vi "Joystick and Camera SHIH V3.2 - external Connection.vi"(7 "Measurement Point":string, 8 "times per measurement":i32, 9 "Motion in":refnum<class "Motion.lvclass">) -> (0 "error out 2":errorcluster, 2 "final out":dbl[](array[numeric]), 3 "Motion out 2":refnum<class "Motion.lvclass">, 4 "GANTRY position":dbl[](array[numeric]), 5 "radius/stddev":dbl[](array[numeric]))   [LabVIEW 2016]
uses:
  Classes/Controllers/Motion/Copy of Motion Folder/Motion.lvclass
  Classes/Controllers/Camera/Copy of Camera Folder/Machine Vision.ctl
  Classes/Controllers/Camera/Copy of Camera Folder/Camera.lvclass
  Classes/Controllers/Camera/Copy of Controller Folder/Controller.lvclass
panel:
  out "loop index":i32
  out "Radius Standard Dev":dbl
  out "Radius  Mean":dbl
  out "Y Standard Dev":dbl
  out "Y Arithmetic Mean":dbl
  out "X Standard Dev":dbl
  out "X Arithmetic Mean":dbl
  out "camera R":dbl
  out "Image 2":T1(plugin-control)
  out "Numeric":dbl
  out "Image":T1(plugin-control)
  out "Camera":dbl[](array[numeric])
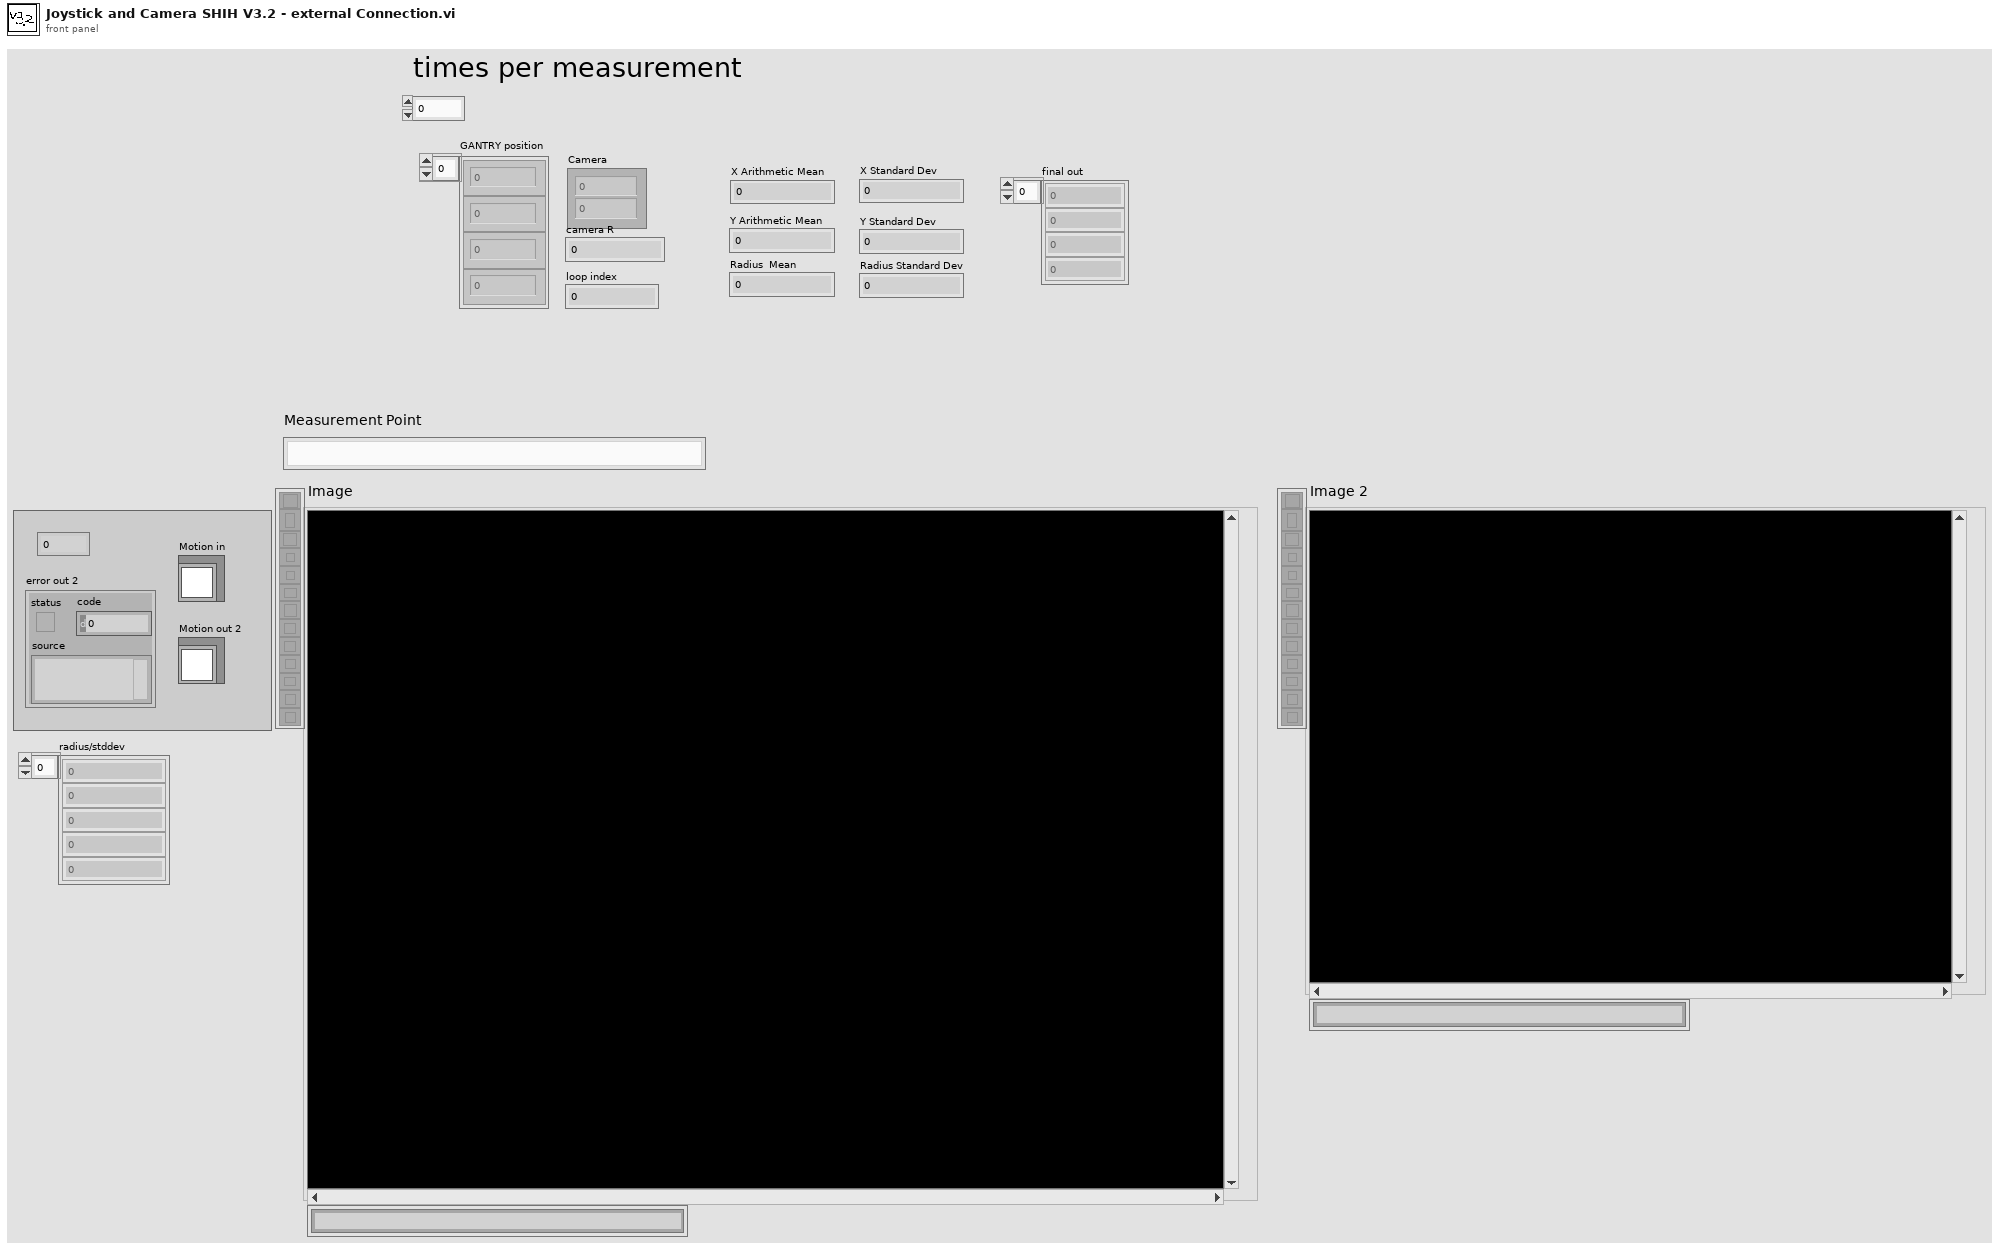
[diagram p1: front panel]
types:
  T1 = typedef "IMAQ Image.ctl" = refnum<image>
  T2 = typedef "Controller.lvclass/Controllers.ctl" = cluster{"Copy of Motion.lvclass":refnum<class "Motion.lvclass">, "Copy of I-O.lvclass":refnum<class "I-O.lvclass">, "Copy of Dispenser.lvclass":refnum<class "Dispenser.lvclass">}
  T3 = typedef "Camera.lvclass/Machine Vision.ctl" = enum16{"Focus", "chip cross", "LargeCircle", "None", "INTT HDI Mark", "INTT Sensor Cross", "INTT Chip Corner", "HPK Silicon", "circle"}
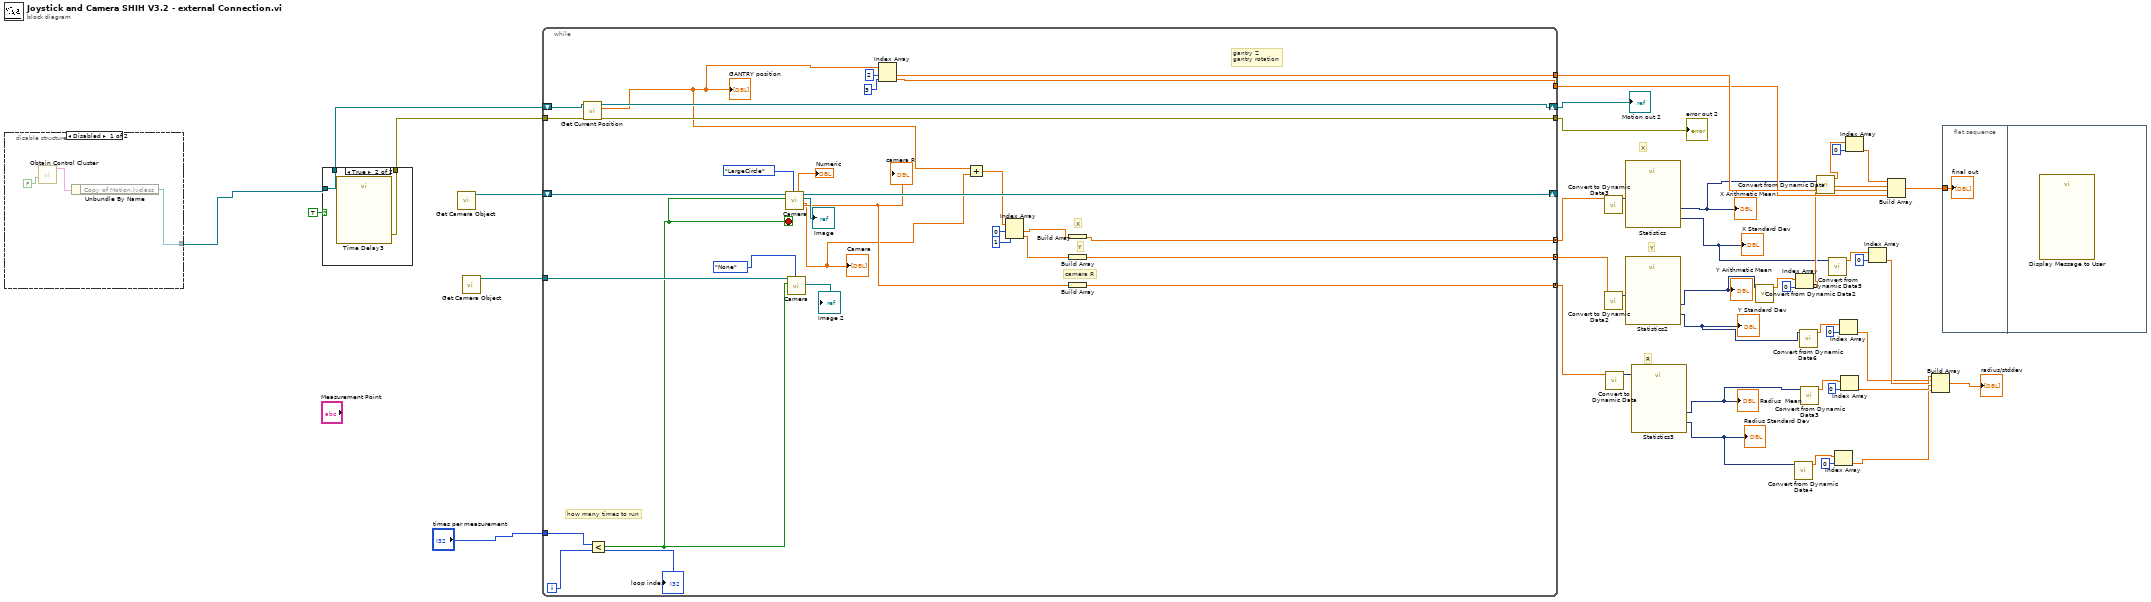
[diagram p0: block diagram]
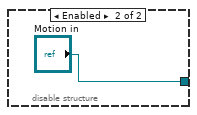
[diagram p2: hidden frame]
diagram:
  # "R"
  # "Y"
  # "X"
  n1 = disable-structure shown="Disabled" {
    disable-tunnel: [w44 "Motion in"] -> w28
    frame Disabled {
      n2 = call "Obtain Control Cluster.vi"("I/O"=FALSE) -> ("Control Out"=w46:T2)  [unwired: 10 in]
      n3 = Unbundle By Name(w46) -> ("Copy of Motion.lvclass"=w44:refnum<class "Motion.lvclass">)
    }
    frame Enabled {
    }
  }
  n4 = case shown="True" TRUE {
    tunnel: [w48 w50] -> w34
    tunnel: w28 -> [w48 w50]
    tunnel: [_ w49] -> w32
    frame False {
    }
    frame True {
      n5 = call "Time Delay3"() -> ("error out"=w49:errorcluster)  [unwired: 11 in]
    }
  }
  n6 = call "Get Camera Object.vi"() -> ("Camera out"=w43:refnum<class "Camera.lvclass">)  [unwired: 10 in, 1 out]
  n7 = call "Get Camera Object.vi"() -> ("Camera out"=w42:refnum<class "Camera.lvclass">)  [unwired: 10 in, 1 out]
  n8 = while {
    shift-right: [w79] -> _
    shift-left: w43 -> [w80]
    tunnel: w42 -> [w76]
    tunnel: [w68] -> w37 mode=concatenating
    tunnel: [w67] -> w39 mode=concatenating
    tunnel: [w66] -> w41 mode=concatenating
    shift-right: [w64] -> w33
    shift-left: w34 -> [w65]
    tunnel: w32 -> [w63]
    tunnel: [w62] -> w31
    tunnel: "times per measurement" -> [w61]
    tunnel: [w55] -> w30
    tunnel: [w54] -> w29
    i -> [w74]
    stop <- w51 stop-if-true
    # "gantry Z\ngantry rotation"
    # "how many times to run"
    # "camera R"
    # "Y"
    # "X"
    n9 = call-dynamic "Get Current Position.vi"("error in (no error)"=w63, "Motion in"=w65) -> ("error out"=w62:errorcluster, "XYZTheta Out"=w58:dbl[], "Motion out"=w64:refnum<class "Motion.lvclass">)  [unwired: 7 in]
    "GANTRY position" <- w58
    n10 = Less?(x=w61, y=w74) -> (x < y?=w51:bool)
    n11 = call "Camera.vi"("Machine Vision"=Machine_Vision."LargeCircle", "Stop"=w51, "Camera in"=w80) -> ("Camera"=w60:dbl[], "Image"=→"Image":T1, "Camera out"=w79:refnum<class "Camera.lvclass">, "Numeric"=→"Numeric":dbl, "camera R"=w73:dbl)  [unwired: 2 in, 2 out]
    "Camera" <- w60
    "camera R" <- w73
    n12 = call "Camera.vi"("Machine Vision"=Machine_Vision."None", "Stop"=w51, "Camera in"=w76) -> ("Image"=→"Image 2":T1)  [unwired: 2 in, 6 out]
    n13 = Index Array(array=w58, index #1=2 ("index"), index #2=3 ("index")) -> (element #1=w55:dbl, element #2=w54:dbl)
    n14 = Add(x=w58, y=w60) -> (x+y=w59:dbl[])
    n15 = Index Array(array=w59, index #1=0 ("index"), index #2=1 ("index")) -> (element #1=w70:dbl, element #2=w69:dbl)
    n16 = Build Array(w70) -> (w68:dbl[])
    n17 = Build Array(w69) -> (w67:dbl[])
    n18 = Build Array(w73) -> (w66:dbl[])
    "loop index" <- w74
  }
  "Motion out 2" <- w33
  "error out 2" <- w31
  n19 = call "Convert to Dynamic Data3"("Array"=w37) -> ("Dynamic Data Type"=w36:dynamicdata)  [unwired: 3 in]
  n20 = call "Convert to Dynamic Data2"("Array"=w39) -> ("Dynamic Data Type"=w38:dynamicdata)  [unwired: 3 in]
  n21 = call "Convert to Dynamic Data"("Array"=w41) -> ("Dynamic Data Type"=w40:dynamicdata)  [unwired: 3 in]
  n22 = call "Statistics"("Signals"=w36) -> ("Standard Dev"=w10:dynamicdata, "Arithmetic Mean"=w27:dynamicdata)  [unwired: 24 in, 1 out]
  "X Arithmetic Mean" <- w27
  "X Standard Dev" <- w10
  n23 = call "Statistics2"("Signals"=w38) -> ("Standard Dev"=w7:dynamicdata, "Arithmetic Mean"=w23:dynamicdata)  [unwired: 24 in, 1 out]
  "Y Arithmetic Mean" <- w23
  "Y Standard Dev" <- w7
  n24 = call "Statistics3"("Signals"=w40) -> ("Standard Dev"=w13:dynamicdata, "Arithmetic Mean"=w16:dynamicdata)  [unwired: 24 in, 1 out]
  "Radius  Mean" <- w16
  "Radius Standard Dev" <- w13
  n25 = call "Convert from Dynamic Data2"("Dynamic Data Type"=w23) -> ("Array"=w24:dbl[])  [unwired: 3 in]
  n26 = call "Convert from Dynamic Data4"("Dynamic Data Type"=w13) -> ("Array"=w14:dbl[])  [unwired: 3 in]
  n27 = Index Array(array=w24, index=0) -> (element=w20:dbl)
  n28 = call "Convert from Dynamic Data6"("Dynamic Data Type"=w7) -> ("Array"=w8:dbl[])  [unwired: 3 in]
  n29 = call "Convert from Dynamic Data3"("Dynamic Data Type"=w16) -> ("Array"=w17:dbl[])  [unwired: 3 in]
  n30 = call "Convert from Dynamic Data"("Dynamic Data Type"=w27) -> ("Array"=w22:dbl[])  [unwired: 3 in]
  n31 = call "Convert from Dynamic Data5"("Dynamic Data Type"=w10) -> ("Array"=w11:dbl[])  [unwired: 3 in]
  n32 = Index Array(array=w14, index=0) -> (element=w2:dbl)
  n33 = Index Array(array=w8, index=0) -> (element=w4:dbl)
  n34 = Index Array(array=w17, index=0) -> (element=w3:dbl)
  n35 = Index Array(array=w22, index=0) -> (element=w21:dbl)
  n36 = Index Array(array=w11, index=0) -> (element=w5:dbl)
  n37 = Build Array(w21, w20, w30, w29) -> (w19:dbl[])
  n38 = Build Array(w5, w4, w3, w2) -> (→"radius/stddev":dbl[])
  n39 = flat-sequence {
    tunnel: w19 -> [w81]
    frame #0 {
      "final out" <- w81
    }
    frame #1 {
      n40 = call "Display Message to User"() -> ()  [unwired: 10 in, 2 out]
    }
  }
